vi "Network-Write Response.vi"(0 "connection ID":refnum<k5>, 7 "TCPMessage":T1={"Code"=200, "Command"="", "Payload"="{}"}, 9 "timeout (ms)":i32=5000, 11 "error in (no error)":errorcluster) -> (4 "connection ID out":refnum<k5>, 15 "error out":errorcluster)   [LabVIEW 2020]
uses:
  Typedefs/Network-TCP Message.ctl
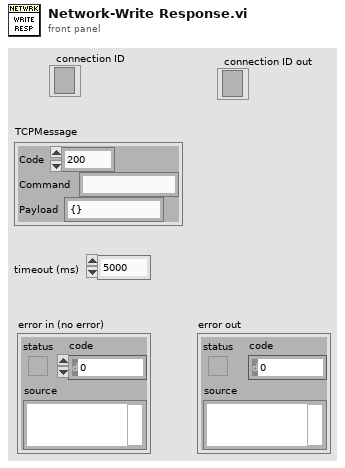
[diagram p1: front panel]
types:
  T1 = typedef "Network-TCP Message.ctl" = cluster{"Code":i32, "Command":string, "Payload":string}
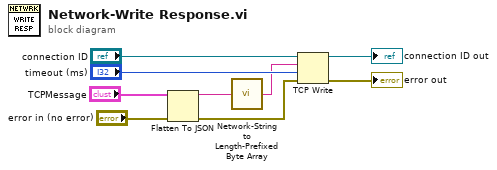
[diagram p0: block diagram]
diagram:
  n1 = Flatten To JSON(anything="TCPMessage", error in (no error)="error in (no error)") -> (JSON string=w3:string, 11:w1:errorcluster)  [unwired: 1 in]
  n2 = call "Network-String to Length-Prefixed Byte Array.vi"("String"=w3) -> ("String"=w7:string)  [unwired: 14 in]
  n3 = TCP Write(connection ID="connection ID", data in=w7, error in (no error)=w1, 9:"timeout (ms)") -> (connection ID out=→"connection ID out":refnum<k5>, error out=→"error out":errorcluster)  [unwired: 1 out]
